vi "Init.vi"(8 "error in (no error)":errorcluster, 11 "Blueprint Qty Event":refnum<user-event>) -> (0 "error out":errorcluster, 3 "BP Summary out":refnum<class "BP Summary.lvclass">)   [LabVIEW 2020, in "BP Summary.lvclass"]
uses:
  BP Summary.lvclass
  App/Blueprint Qty.ctl
  Blueprint/Blueprint.lvclass
  BP Summary.lvclass/BP Summary.ctl
  App/App.lvclass
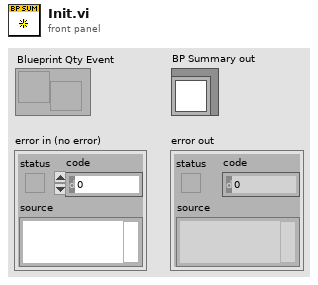
[diagram p1: front panel]
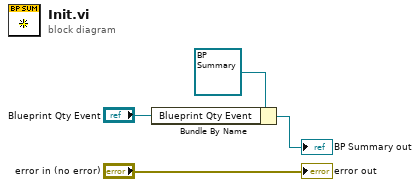
[diagram p0: block diagram]
diagram:
  n1 = Bundle By Name(cluster=refnum<class "BP Summary.lvclass"> refnum ("BP Summary in"), "Blueprint Qty Event"="Blueprint Qty Event") -> (→"BP Summary out":refnum<class "BP Summary.lvclass">)
  "error out" <- "error in (no error)"
